vi "Demodulate.vi"(8 "error in (no error)":errorcluster, 10 "Data in":dbl[](array[numeric]), 11 "Software Lock-in in":refnum<class "Software Lock-in.lvclass">) -> (0 "error out":errorcluster, 2 "Filtered Data":cdb[](array[numeric]), 3 "Software Lock-in out":refnum<class "Software Lock-in.lvclass">)   [LabVIEW 2015, in "Software Lock-in.lvclass"]
uses:
  Software Lock-in.lvclass
  Software Lock-in.lvclass/Software Lock-in.ctl
  <vilib>/Analysis/2dsp.llb/Decimate (continuous, CDB).vi
  <vilib>/Analysis/3filter.llb/IIR Filter (CDB).vi
  <vilib>/Analysis/NI_AALPro.lvlib
  <vilib>/Analysis/NI_AALBase.lvlib
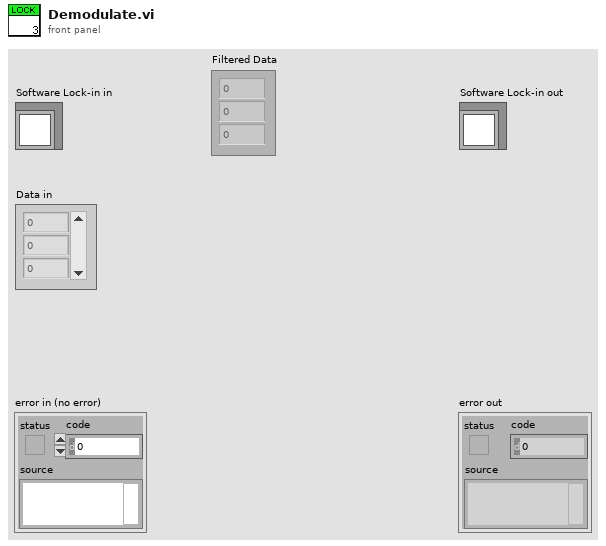
[diagram p1: front panel]
types:
  T1 = typedef "Lock-in modulation.ctl" = cdb[]
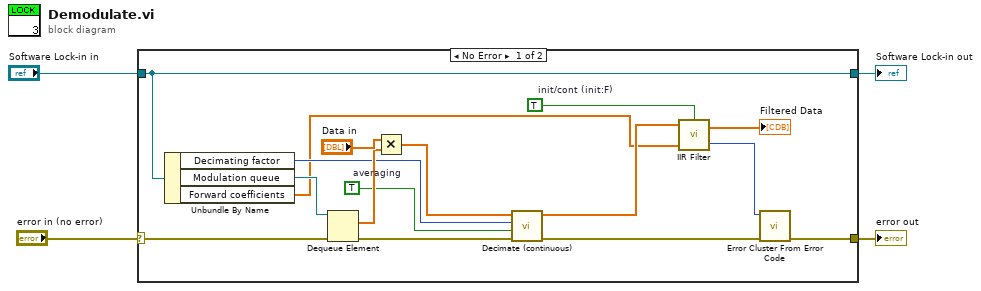
[diagram p0: block diagram]
diagram:
  n1 = case shown="No Error" "error in (no error)" {
    selector: "error in (no error)" -> [w18 w22]
    tunnel: [w6 w22] -> w3
    tunnel: [w20 w21] -> w1
    tunnel: "Software Lock-in in" -> [w20 w21]
    frame No Error {
      w11 = TRUE  # init/cont (init:F)
      w14 = TRUE  # averaging
      n2 = Unbundle By Name(w20) -> ("Decimating factor"=w13:i32, "Modulation queue"=w19:refnum<queue>, "Forward coefficients"=w10:dbl[])
      n3 = Dequeue Element(queue=w19, error in (no error)=w18) -> (element=w16:T1, error out=w7:errorcluster)  [unwired: 1 in, 2 out]
      n4 = Multiply(x="Data in", y=w16) -> (x*y=w15:T1)
      n5 = call-poly <vilib>:"Decimate (continuous).vi"("error in (no error)"=w7, "averaging"=w14, "decimating factor"=w13, "X"=w15) -> ("error out"=w8:errorcluster, "Decimated Array"=w12:cdb[])  [unwired: 6 in]
      n6 = call-poly <vilib>:"IIR Filter.vi"("init/cont (init:F)"=w11, "Forward Coefficients"=w10, "X"=w12) -> ("error"=w9:i32, "Filtered X"=→"Filtered Data":cdb[])  [unwired: 1 in]
      n7 = call <vilib>:"Error Cluster From Error Code.vi"("error in (no error)"=w8, "error code (0)"=w9) -> ("error out"=w6:errorcluster)  [unwired: 7 in]
    }
    frame Error {
    }
  }
  "error out" <- w3
  "Software Lock-in out" <- w1
